vi "ClosePiezo.vi"(8 "error in (no error)":errorcluster, 9 "MG17 X":refnum<k7>, 10 "MG17 Z":refnum<k7>, 11 "MG17 Y":refnum<k7>) -> (0 "error out":errorcluster)   [LabVIEW 2014]
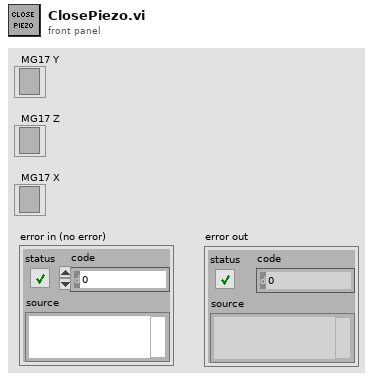
[diagram p1: front panel]
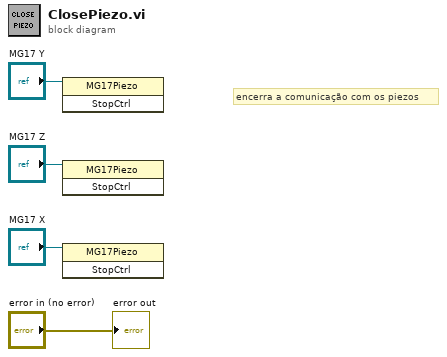
[diagram p0: block diagram]
diagram:
  # "encerra a comunicação com os piezos"
  n1 = invoke class="MG17Piezo" method="StopCtrl"(reference="MG17 Y") -> ()  [unwired: 2 in, 3 out]
  n2 = invoke class="MG17Piezo" method="StopCtrl"(reference="MG17 Z") -> ()  [unwired: 2 in, 3 out]
  n3 = invoke class="MG17Piezo" method="StopCtrl"(reference="MG17 X") -> ()  [unwired: 2 in, 3 out]
  "error out" <- "error in (no error)"
